vi "RW All Data.vi"(2 "R/W Case":T1, 7 "RT Data in":T2={"Device ref"=0, "Scan Period (uSec)"=10000, "Device Channels"={"Status"={"BD Refs"=[], "Length"=0, "FIFO Index"=0, "Data"=[]}, "Command"={"BD Refs"=[], "Data"=[], "Length"=0, "FIFO Index"=0}}, "Local Chassis"=[], "EtherCAT Masters"=[], "Async"={"Status"=refnum, "Command"=refnum, "Input FIFO"=refnum, "Input FIFO buffer"=[], "Output FIFO"=refnum, "Output FIFO buffer"=[], "Async VI Ref"=refnum}, "ECAT Reconfig"={"Reconfig Module Found"=FALSE, "VI Ref"=refnum, "Status"=refnum}, "Device Error"={"status"=FALSE, "code"=0, "source"=""}, "DeviceName"="", "PCLSync?"=FALSE} {"Device Channels"."Status"."BD Refs"."Data Reference" format="%.0x"; "Device Channels"."Command"."BD Refs"."Data Reference" format="%.0x"; "Local Chassis"."FPGA"."VS ref" format="%.0x"; "Local Chassis"."RSI Modules"."VS ref" format="%.0x"; "Local Chassis"."VS ref" format="%.0x"; "Device ref" format="%.0x"; "EtherCAT Masters"."REM IO ECAT Slaves"."VS ref" format="%.0x"; "EtherCAT Masters"."Generic EtherCAT Slaves"."VS ref" format="%.0x"; "EtherCAT Masters"."VS ref" format="%.0x"; "EtherCAT Masters"."EtherCAT Slaves"."FPGA"."VS ref" format="%.0x"; "EtherCAT Masters"."EtherCAT Slaves"."RSI Modules"."VS ref" format="%.0x"; "EtherCAT Masters"."EtherCAT Slaves"."VS ref" format="%.0x"}) -> (8 "RT Data out":T2={"Device ref"=0, "Scan Period (uSec)"=10000, "Device Channels"={"Status"={"BD Refs"=[], "Length"=0, "FIFO Index"=0, "Data"=[]}, "Command"={"BD Refs"=[], "Data"=[], "Length"=0, "FIFO Index"=0}}, "Local Chassis"=[], "EtherCAT Masters"=[], "Async"={"Status"=refnum, "Command"=refnum, "Input FIFO"=refnum, "Input FIFO buffer"=[], "Output FIFO"=refnum, "Output FIFO buffer"=[], "Async VI Ref"=refnum}, "ECAT Reconfig"={"Reconfig Module Found"=FALSE, "VI Ref"=refnum, "Status"=refnum}, "Device Error"={"status"=FALSE, "code"=0, "source"=""}, "DeviceName"="", "PCLSync?"=FALSE} {"Device Channels"."Status"."BD Refs"."Data Reference" format="%.0x"; "Device Channels"."Command"."BD Refs"."Data Reference" format="%.0x"; "Local Chassis"."FPGA"."VS ref" format="%.0x"; "Local Chassis"."RSI Modules"."VS ref" format="%.0x"; "Local Chassis"."VS ref" format="%.0x"; "Device ref" format="%.0x"; "EtherCAT Masters"."REM IO ECAT Slaves"."VS ref" format="%.0x"; "EtherCAT Masters"."Generic EtherCAT Slaves"."VS ref" format="%.0x"; "EtherCAT Masters"."VS ref" format="%.0x"; "EtherCAT Masters"."EtherCAT Slaves"."FPGA"."VS ref" format="%.0x"; "EtherCAT Masters"."EtherCAT Slaves"."RSI Modules"."VS ref" format="%.0x"; "EtherCAT Masters"."EtherCAT Slaves"."VS ref" format="%.0x"})   [LabVIEW 2020, in "SEECD Engine.lvlib"]
uses:
  SEECD Engine.lvlib
  <vilib>/NI VeriStand/Custom Device API/Custom Device Item Ref.ctl
  <vilib>/NI VeriStand/Custom Device API/Custom Device API.lvlib
  Includes/Modules.lvlibp/RSI Module/RSI Module.lvclass
  <vilib>/NI VeriStand/Custom Device API/Data Reference.ctl
  <vilib>/NI VeriStand/Custom Device API/Block Data Reference.ctl
  Type Defs/Input Data.ctl
  Type Defs/Output Data.ctl
  Type Defs/RSI Module Data.ctl
  Type Defs/FPGA Data.ctl
  Type Defs/EtherCAT Slave Data.ctl
  Type Defs/EtherCAT Master Data.ctl
  Type Defs/Local Chassis Data.ctl
  Type Defs/RT Data.ctl
  Includes/Modules.lvlibp/RSI Module/Channel Type.ctl
  Type Defs/Async Command.ctl
  Type Defs/Async Status.ctl
  Type Defs/Async State.ctl
  Type Defs/RW Case.ctl
  Shared/Type Defs/UDV Data Type.ctl
  Shared/SEECD Shared.lvlib
  Shared/Type Defs/FXP Config.ctl
  Type Defs/UDV Data.ctl
  Includes/Modules.lvlibp/RSI Module/Module Models.ctl
  Type Defs/Module Config Data.ctl
  Type Defs/Async Data.ctl
  Type Defs/ECAT Reconfig State.ctl
  Type Defs/ECAT Reconfig Status.ctl
  Type Defs/ECAT Reconfig Data.ctl
  Type Defs/Device Channels.ctl
  Type Defs/Mixed IO.ctl
  Type Defs/Open Module IOVs.ctl
  Type Defs/Mod Size Indexes.ctl
  Type Defs/Generic ECAT Slave IOV Cluster.ctl
  Type Defs/Generic ECAT Slave Data Cluster.ctl
  Type Defs/Generic ECAT Slave RT-Data-Array.ctl
  Type Defs/REM IO ECAT Slave IOV Cluster.ctl
  Type Defs/REM IO ECAT Slave Data Cluster.ctl
  Type Defs/REM IO ECAT Slave RT-Data-Array.ctl
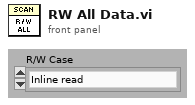
[diagram p1: front panel]
types:
  T1 = typedef "SEECD Engine.lvlib/RW Case.ctl" = enum16{"Inline read", "Inline write", "Async - Inline loop read", "Async - Inline loop write", "Async loop (read/write)"}
  T2 = typedef "SEECD Engine.lvlib/RT Data.ctl" = cluster{"Device ref":T3, "Scan Period (uSec)":u32, "Device Channels":T4, "Local Chassis":T9[], "EtherCAT Masters":T21[], "Async":T29, "ECAT Reconfig":T30, "Device Error":errorcluster, "DeviceName":string, "PCLSync?":bool}
  T3 = typedef "Custom Device API.lvlib/Custom Device Item Ref.ctl" = u64
  T4 = typedef "SEECD Engine.lvlib/Device Channels.ctl" = cluster{"Status":T5, "Command":T8}
  T5 = typedef "SEECD Engine.lvlib/Output Data.ctl" = cluster{"BD Refs":T6[], "Length":i32, "FIFO Index":i32, "Data":dbl[]}
  T6 = typedef "Custom Device API.lvlib/Block Data Reference.ctl" = cluster{"Data Reference":T7, "Offset":u64, "Length":u64}
  T7 = typedef "Custom Device API.lvlib/Data Reference.ctl" = i32
  T8 = typedef "SEECD Engine.lvlib/Input Data.ctl" = cluster{"BD Refs":T6[], "Data":dbl[], "Length":i32, "FIFO Index":i32}
  T9 = typedef "SEECD Engine.lvlib/Local Chassis Data.ctl" = cluster{"VS ref":T3, "RSI Modules":T10[], "FPGA":T16[], "Input Mod Size Idxs":T20, "Output Modules":i32[], "MixedIO Mod Size Idxs":T20}
  T10 = typedef "SEECD Engine.lvlib/RSI Module Data.ctl" = cluster{"VS ref":T3, "IOV ref":refnum<k21>, "Open Mod refs":T11, "Module DVR":refnum<data-value>, "Slot":u32, "Model":T12, "Channel Type":T13, "EtherCAT?":bool, "CDInput Data":T8, "CDOutput Data":T5, "Module Config Data":T14, "Mixed IO":T15}
  T11 = typedef "SEECD Engine.lvlib/Open Module IOVs.ctl" = cluster{"Analog Read":refnum<k21>, "Digital Read":refnum<k21>, "Analog Write":refnum<k21>, "Digital Write":refnum<k21>}
  T12 = typedef "Modules.lvlibp/RSI Module.lvclass/Module Models.ctl" = enum16{"Empty", "NI 9201", "NI 9203", "NI 9205", "NI 9206", "NI 9207", "NI 9208", "NI 9209", "NI 9210", "NI 9211", "NI 9212", "NI 9213", "NI 9214", "NI 9215", "NI 9216", "NI 9217", "NI 9219", "NI 9220", "NI 9221", "NI 9222", "NI 9223", "NI 9224", "NI 9225", "NI 9226", "NI 9227", "NI 9228", "NI 9229", "NI 9233", "NI 9234", "NI 9235", "NI 9236", "NI 9237", "NI 9239", "NI 9242", "NI 9244", "NI 9253", "NI 9263", "NI 9264", "NI 9265", "NI 9266", "NI 9269", "NI 9344", "NI 9350", "NI 9375", "NI 9401", "NI 9402", "NI 9403", "NI 9411", "NI 9421", "NI 9422", "NI 9423", "NI 9425", "NI 9426", "NI 9435", "NI 9436", "NI 9437", "NI 9472", "NI 9474", "NI 9475", "NI 9476", "NI 9477", "NI 9478", "NI 9481", "NI 9482", "NI 9485"}
  T13 = typedef "Modules.lvlibp/RSI Module.lvclass/Channel Type.ctl" = enum16{"Analog", "Digital"}
  T14 = typedef "SEECD Engine.lvlib/Module Config Data.ctl" = cluster{"Configurable?":bool, "Config Block Data Refs":T6[], "Config Data DVR":refnum<data-value>, "Previous Values":dbl[], "Local Reconfig VI Ref":refnum<vi>}
  T15 = typedef "SEECD Engine.lvlib/Mixed IO.ctl" = cluster{"Input Channel Indices":i32[], "Input Buffer":dbl[]}
  T16 = typedef "SEECD Engine.lvlib/FPGA Data.ctl" = cluster{"VS ref":T3, "IOV ref":refnum<k21>, "FPGA Target":enum16{"Local", "EtherCAT"}, "Product Code":u32, "Bitfile Signature":string, "Bitfile Path (RT)":path, "FPGA Session":u32, "Input Data":T8, "Output Data":T5, "UDVs":cluster{"From FPGA":T17[], "To FPGA":T17[]}}
  T17 = typedef "SEECD Engine.lvlib/UDV Data.ctl" = cluster{"VS ref":T3, "IOV Ref":refnum<k21>, "Name":string, "UDV Data Type":T18, "Supported Type?":bool, "FXP Config":T19, "FXP VI Ref":refnum<vi>}
  T18 = typedef "SEECD Shared.lvlib/UDV Data Type.ctl" = enum16{"Boolean", "Fixed Point", "Int8", "Int16", "Int32", "Int64", "U32 Bit Field", "UInt8", "UInt16", "UInt32", "UInt64", "Other", "DBL", "SGL"}
  T19 = typedef "SEECD Shared.lvlib/FXP Config.ctl" = cluster{"signed":bool, "size":u32, "integersize":i32}
  T20 = typedef "SEECD Engine.lvlib/Mod Size Indexes.ctl" = cluster{"4":i32[], "8":i32[], "16":i32[], "32":i32[], "other":i32[]}
  T21 = typedef "SEECD Engine.lvlib/EtherCAT Master Data.ctl" = cluster{"VS ref":T3, "IOV ref":refnum<k21>, "Master ID":u32, "Cyclic Data Bandwidth":u32, "EtherCAT Slaves":T22[], "Generic EtherCAT Slaves":T23, "REM IO ECAT Slaves":T26}
  T22 = typedef "SEECD Engine.lvlib/EtherCAT Slave Data.ctl" = cluster{"VS ref":T3, "IOV ref":refnum<k21>, "Position Address":u16, "RSI Modules":T10[], "FPGA":T16[], "Input Mod Size Idxs":T20, "Output Modules":i32[], "MixedIO Mod Size Idxs":T20}
  T23 = typedef "SEECD Engine.lvlib/Generic ECAT Slave RT-Data-Array.ctl" = T24[]
  T24 = typedef "SEECD Engine.lvlib/Generic ECAT Slave Data Cluster.ctl" = cluster{"VS ref":T3, "IOV ref":refnum<k21>, "Position Address":u16, "I/O Imput Vars ":T25[], "I/O Output Vars":T25[], "I/O Input Data":T8, "I/O Output Data":T5, "Distributed Clock":bool}
  T25 = typedef "SEECD Engine.lvlib/Generic ECAT Slave IOV Cluster.ctl" = cluster{"VS ref":T3, "IOV Ref":refnum<k21>, "Name":string, "UDV Data Type":T18}
  T26 = typedef "SEECD Engine.lvlib/REM IO ECAT Slave RT-Data-Array.ctl" = T27[]
  T27 = typedef "SEECD Engine.lvlib/REM IO ECAT Slave Data Cluster.ctl" = cluster{"VS ref":T3, "IOV ref":refnum<k21>, "Position Address":u16, "I/O Imput Vars ":T28[], "I/O Output Vars":T28[], "I/O Input Data":T8, "I/O Output Data":T5}
  T28 = typedef "SEECD Engine.lvlib/REM IO ECAT Slave IOV Cluster.ctl" = cluster{"VS ref":T3, "IOV Ref":refnum<k21>, "Name":string, "UDV Data Type":T18, "Scaling Factor":dbl}
  T29 = typedef "SEECD Engine.lvlib/Async Data.ctl" = cluster{"Status":refnum<queue>, "Command":refnum<queue>, "Input FIFO":refnum<k33>, "Input FIFO buffer":dbl[], "Output FIFO":refnum<k33>, "Output FIFO buffer":dbl[], "Async VI Ref":refnum<vi>}
  T30 = typedef "SEECD Engine.lvlib/ECAT Reconfig Data.ctl" = cluster{"Reconfig Module Found":bool, "VI Ref":refnum<vi>, "Status":refnum<queue>}
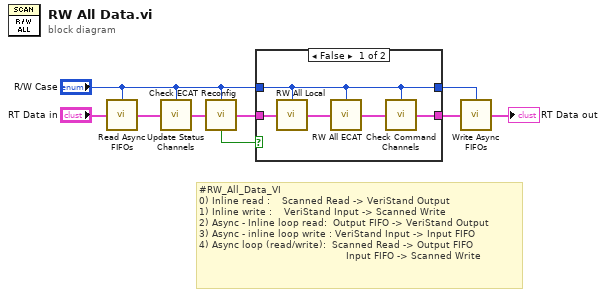
[diagram p0: block diagram]
diagram:
  # "#RW_All_Data_VI\n0) Inline read\t:\t\t\t\tScanned Read -> VeriStand Output\n1) Inline write\t:\t\t\t\tVeriStand Input -> Scanned Write\n2) Async - Inline loop read:\t\tOutput FIFO -> VeriStand Output\n3) Async - inline loop write\t: VeriStand Input -> Input FIFO\n4) Async loop (read/write):\t\tScanned Read -> Output FIFO\n\t\t\t\t\t                                            Input FIFO -> Scanned Write"
  n1 = call "Read Async FIFOs.vi"("R/W Case"="R/W Case", "RT Data in"="RT Data in") -> ("RT Data out"=w7:T2)  [unwired: 13 in]
  n2 = call "Update Status Channels.vi"("R/W Case"="R/W Case", "RT Data in"=w7) -> ("RT Data out"=w6:T2)  [unwired: 13 in]
  n3 = call "Check ECAT Reconfig.vi"("R/W Case"="R/W Case", "RT Data in"=w6) -> ("RT Data out"=w4:T2, "ECAT Reconfig?"=w5:bool)  [unwired: 12 in]
  n4 = case shown="False" w5 {
    tunnel: "R/W Case" -> [w11 w16]
    tunnel: [w11 w16] -> w2
    tunnel: w4 -> [w14 w15]
    tunnel: [w10 w15] -> w3
    frame False {
      n5 = call "RW All Local.vi"("R/W Case"=w11, "RT Data in"=w14) -> ("RT Data out"=w13:T2)  [unwired: 13 in]
      n6 = call "RW All ECAT.vi"("R/W Case"=w11, "RT Data in"=w13) -> ("RT Data out"=w12:T2)  [unwired: 13 in]
      n7 = call "Check Command Channels.vi"("R/W Case"=w11, "RT Data in"=w12) -> ("RT Data out"=w10:T2)  [unwired: 13 in]
    }
    frame True {
    }
  }
  n8 = call "Write Async FIFOs.vi"("R/W Case"=w2, "RT Data in"=w3) -> ("RT Data out"=→"RT Data out":T2)  [unwired: 13 in]
